vi "Read Date Yields.vi"(8 "error in (no error)":errorcluster, 11 "Master in":refnum<class "Master.lvclass">) -> (0 "error out":errorcluster, 3 "Master out":refnum<class "Master.lvclass">)   [LabVIEW 2014, in "Master.lvclass"]
uses:
  Master/Master.lvclass
  Master/Master.lvclass/Master.ctl
panel:
  in  "Production":T1
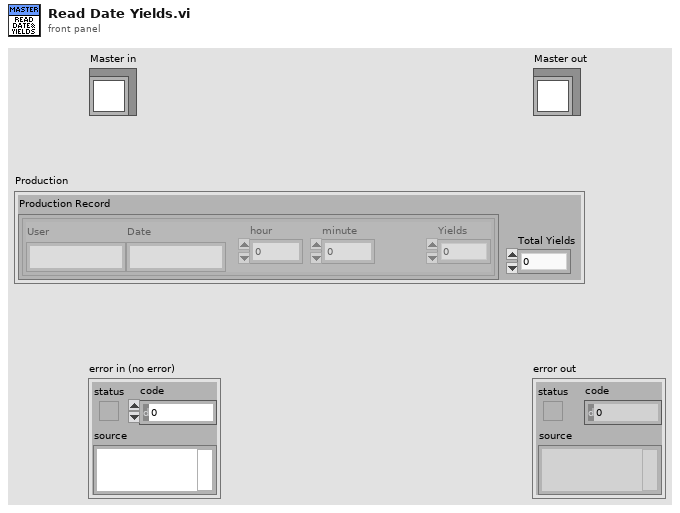
[diagram p1: front panel]
types:
  T1 = cluster{"Production Record":cluster{"User":string, "Date":string, "Yields":dbl, "hour":i32, "minute":i32}[], "Total Yields":dbl}
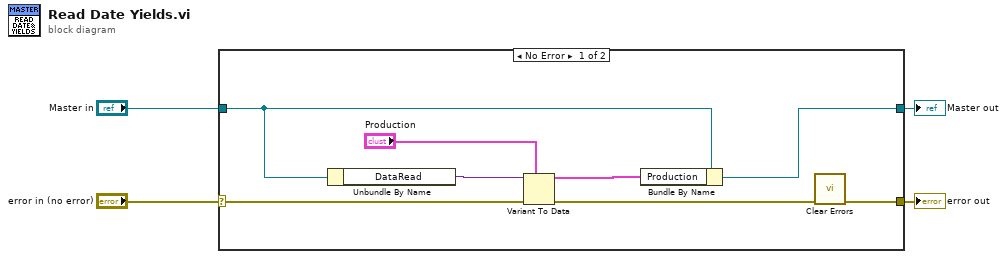
[diagram p0: block diagram]
diagram:
  n1 = case shown="No Error" "error in (no error)" {
    selector: "error in (no error)" -> [w8 w14]
    tunnel: [w5 w14] -> w3
    tunnel: [w10 w13] -> w1
    tunnel: "Master in" -> [w9 w13]
    frame No Error {
      n2 = Unbundle By Name(w9) -> ("DataRead"=w11:variant)
      n3 = Variant To Data(error in=w8, type="Production", Variant=w11) -> (data=w12:T1, error out=w6:errorcluster)
      n4 = Bundle By Name(cluster=w9, "Production"=w12) -> (w10:refnum<class "Master.lvclass">)
      n5 = call <vilib>:"Clear Errors.vi"("error in (no error)"=w6) -> ("error out"=w5:errorcluster)  [unwired: 5 in, 1 out]
    }
    frame Error {
    }
  }
  "error out" <- w3
  "Master out" <- w1
